vi "from string.vi"(8 "error in":errorcluster, 9 "data":string, 10 "version":string, 11 "module configuration in":refnum<class "fixed channel tag bus module configuration.lvclass">) -> (0 "error out":errorcluster, 3 "module configuration out":refnum<class "fixed channel tag bus module configuration.lvclass">)   [LabVIEW 2013, in "fixed channel tag bus module configuration.lvclass"]
doc: "Provides an interface for loading a module configuration from a file or other serialized data source. It is recommended that all children of this class store data in two sets--data required for its own initialization, and any data required for parent initialization--and that each implementation uses the <b>Call Parent Method</b> primitive to de-serialize parent information. As a result, it is expected that every module configuration class calls <b>component configuration.lvclass:From String.vi</b>.\nNI Tag Bus Module Framework 1.0.3.43\nNI Systems Engineering"
uses:
  fixed channel tag bus module configuration.lvclass
  <vilib>/NI/Tag Bus Module Framework/module configuration/TBM module configuration.lvclass
  <vilib>/NI/Tag Bus Module Framework/channel/TBM channel.lvclass
  fixed channel tag bus module configuration.lvclass/fixed channel tag bus module configuration.ctl
  <vilib>/NI/Tag Bus Module Framework/root configuration/TBM configuration.lvclass
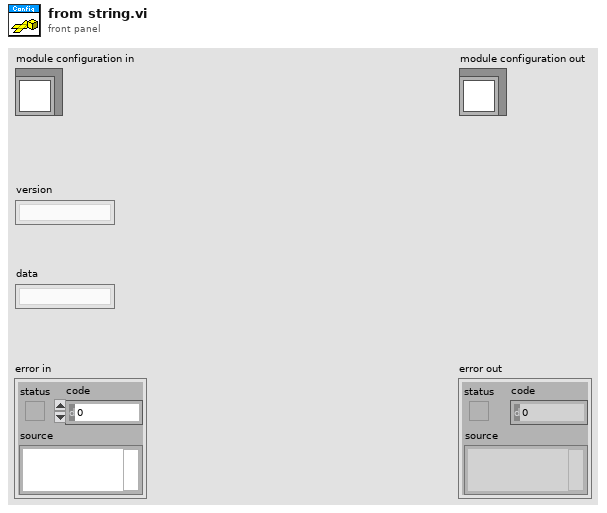
[diagram p1: front panel]
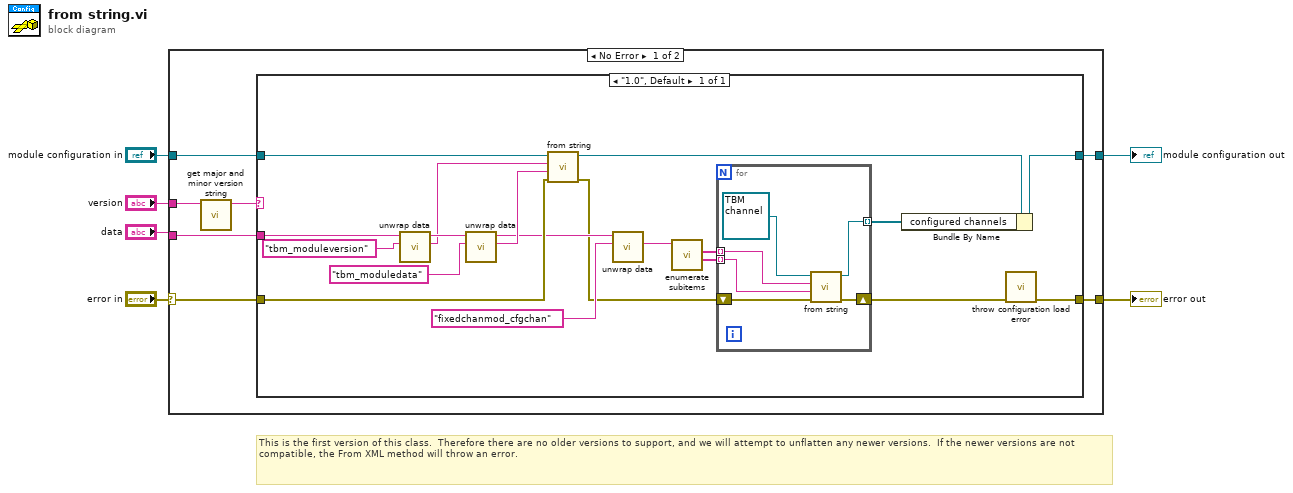
[diagram p0: block diagram]
diagram:
  # "This is the first version of this class.  Therefore there are no older versions to support, and we will attempt to unflatten any newer versions.  If the newer versions are not compatible, the From XML method will throw an error."
  n1 = case shown="No Error" "error in" {
    selector: "error in" -> [w7 w40]
    tunnel: "data" -> [w13 _]
    tunnel: "module configuration in" -> [w12 w39]
    tunnel: [w11 w39] -> w5
    tunnel: [w10 w40] -> w4
    tunnel: "version" -> [w9 _]
    frame No Error {
      n2 = call <vilib>:"get major and minor version string.vi"("full version"=w9) -> ("major.minor version"=w8:string)  [unwired: 10 in]
      n3 = case shown="\"1.0\", Default" w8 {
        tunnel: w13 -> [w31]
        tunnel: w7 -> [w23]
        tunnel: w12 -> [w32]
        tunnel: [w22] -> w11
        tunnel: [w24] -> w10
        frame "1.0", Default {
          n4 = call <vilib>:"unwrap data.vi"("identifier"="tbm_moduleversion" ("additional identifier"), "data to unwrap"=w31) -> ("unwrapped data"=w25:string, "remaining string"=w27:string)  [unwired: 8 in]
          n5 = call <vilib>:"unwrap data.vi"("identifier"="tbm_moduledata" ("additional identifier"), "data to unwrap"=w27) -> ("unwrapped data"=w26:string, "remaining string"=w20:string)  [unwired: 8 in]
          n6 = call-parent "from string.vi"("error in"=w23, "data"=w26, "version"=w25, "module configuration in"=w32) -> ("error out"=w18:errorcluster, "module configuration out"=w30:refnum<class "fixed channel tag bus module configuration.lvclass">)  [unwired: 6 in]
          n7 = call <vilib>:"unwrap data.vi"("identifier"="fixedchanmod_cfgchan", "data to unwrap"=w20) -> ("unwrapped data"=w19:string)  [unwired: 8 in, 1 out]
          n8 = call <vilib>:"enumerate subitems.vi"("data to enumerate"=w19) -> ("associated data"=w15:string[], "discovered subitems"=w16:string[])  [unwired: 8 in, 1 out]
          n9 = for {
            shift-right: [w38] -> w17
            shift-left: w18 -> [w37]
            tunnel: w16 -> [w35] mode=indexing
            tunnel: w15 -> [w34] mode=indexing
            tunnel: [w36] -> w14 mode=indexing
            n10 = call-dynamic "from string.vi"("error in"=w37, "channel data"=w34, "identifier"=w35, "channel in"=refnum<class "TBM channel.lvclass"> refnum) -> ("error out"=w38:errorcluster, "channel out"=w36:refnum<class "TBM channel.lvclass">)  [unwired: 6 in]
          }
          n11 = Bundle By Name(cluster=w30, "configured channels"=w14) -> (w22:refnum<class "fixed channel tag bus module configuration.lvclass">)
          n12 = call <vilib>:"throw configuration load error.vi"("error in"=w17) -> ("error out"=w24:errorcluster)  [unwired: 10 in]
        }
      }
    }
    frame Error {
    }
  }
  "error out" <- w4
  "module configuration out" <- w5
